vi "globalSetUp.vi"(8 "error in (no error)":errorcluster, 11 "Test_Blob in":refnum<class "Test_Blob.lvclass">) -> (0 "error out":errorcluster, 3 "Test_Blob out":refnum<class "Test_Blob.lvclass">)   [LabVIEW 2015, in "Test_Blob.lvclass"]
uses:
  Test_Blob.lvclass
  Global Parameters.vi
  <vilib>/addons/_JKI Toolkits/VI Tester/TestCase.llb/TestCase.lvclass
  _shared/_Unit Tests Shared.lvlib
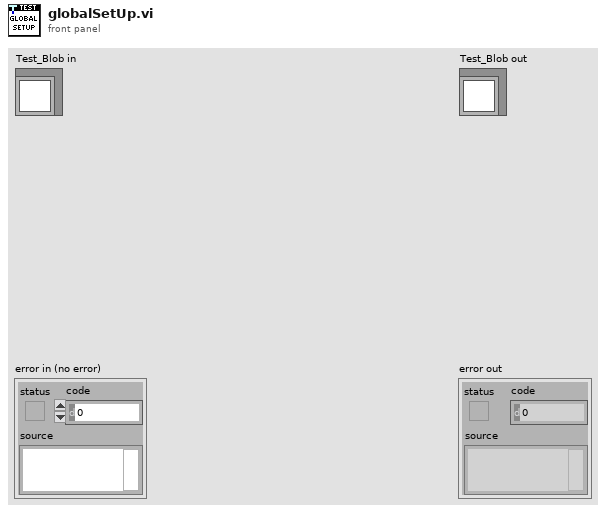
[diagram p1: front panel]
types:
  T1 = typedef "NI_Azure_Core.lvlib/Session.lvclass/Azure Credentials.ctl" = cluster{"Storage Account Name":string, "Access Key":string}
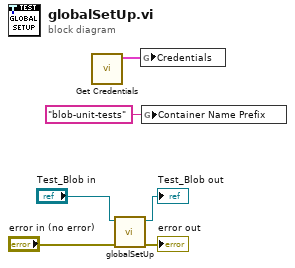
[diagram p0: block diagram]
diagram:
  n1 = call "Get Credentials.vi"() -> ("Azure Credentials"=w2:T1)  [unwired: 11 in]
  n2 = call-parent "globalSetUp.vi"("error in (no error)"="error in (no error)", "TestCase in"="Test_Blob in") -> ("error out"=→"error out":errorcluster, "TestCase out"=→"Test_Blob out":refnum<class "Test_Blob.lvclass">)  [unwired: 8 in]
  n3 = global write "Global Parameters.vi" "Credentials"(w2) -> ()
  n4 = global write "Global Parameters.vi" "Container Name Prefix"("blob-unit-tests" ("Container Name Prefix")) -> ()
